vi "Write DIO Channel Setting.vi"(8 "error in (no error)":errorcluster, 10 "FPGA Channel Setting":T1, 11 "Channel configuration in":refnum<class "Digital IO Channel configuration.lvclass">) -> (0 "error out":errorcluster, 3 "Channel configuration out":refnum<class "Digital IO Channel configuration.lvclass">)   [LabVIEW 2025, in "Digital IO.lvlib" / "Digital IO Channel configuration.lvclass"]
uses:
  Digital IO Channel configuration.lvclass
  DIO Channel Setting.ctl
  Digital IO Channel configuration.lvclass/Digital IO Channel configuration.ctl
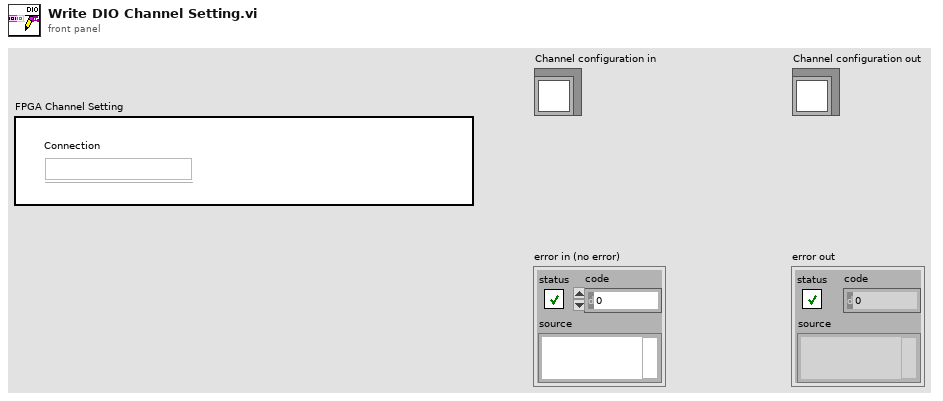
[diagram p1: front panel]
types:
  T1 = typedef "Digital IO.lvlib/Digital IO Channel configuration.lvclass/DIO Channel Setting.ctl" = cluster{"Connection":string}
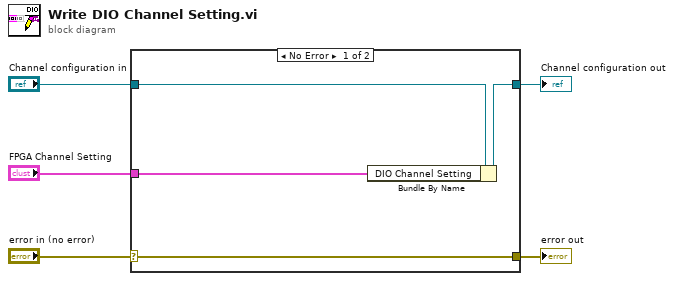
[diagram p0: block diagram]
diagram:
  n1 = case shown="No Error" "error in (no error)" {
    selector: "error in (no error)" -> [w9 w10]
    tunnel: [w9 w10] -> w4
    tunnel: [w7 w11] -> w2
    tunnel: "Channel configuration in" -> [w8 w11]
    tunnel: "FPGA Channel Setting" -> [w6 _]
    frame No Error {
      n2 = Bundle By Name(cluster=w8, "DIO Channel Setting"=w6) -> (w7:refnum<class "Digital IO Channel configuration.lvclass">)
    }
    frame Error {
    }
  }
  "error out" <- w4
  "Channel configuration out" <- w2
